vi "Poll Blowers.vi"(8 "error in (no error)":errorcluster, 11 "cRIO-CO2 in":refnum<class "cRIO-CO2.lvclass">) -> (0 "error IO":errorcluster)   [LabVIEW 2015, in "cRIO-Carbondioxide.lvlib" / "cRIO-CO2.lvlib" / "cRIO-CO2.lvclass"]
uses:
  cRIO-CO2.lvclass
  <vilib>/ActorFramework/Actor/Actor.lvclass/Actor.ctl
  <vilib>/ActorFramework/Message Enqueuer/Message Enqueuer.lvclass/Message Enqueuer.ctl
  Blowers Heaters Enumerator.ctl
  cRIO-CO2 Messages/Launch Blower Msg/Launch Blower Msg.lvclass/Launch Blower Msg.ctl
  <vilib>/ActorFramework/Message Enqueuer/Enqueue.vi
  <vilib>/ActorFramework/Message Enqueuer/Init from Existing Queue.vi
  <vilib>/ActorFramework/Message Priority Queue/Priority Enqueue.vi
  cRIO-CO2 Messages/Launch Blower Msg/Launch Blower Msg.lvclass
  <vilib>/ActorFramework/Message Enqueuer/Message Enqueuer.lvclass
  <vilib>/ActorFramework/Actor/Actor.lvclass
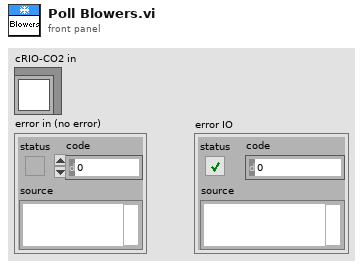
[diagram p1: front panel]
types:
  T1 = typedef "cRIO-Carbondioxide.lvlib/cRIO-CO2.lvlib/cRIO-CO2.lvclass/Blowers Heaters Enumerator.ctl" = enum16{"Tank Blower 1", "Tank Blower 2", "Tank Blower 3", "Tank Blower 4", "Syringe Blower", "Syringe Heater", "Piston Heater", "Undefined"}
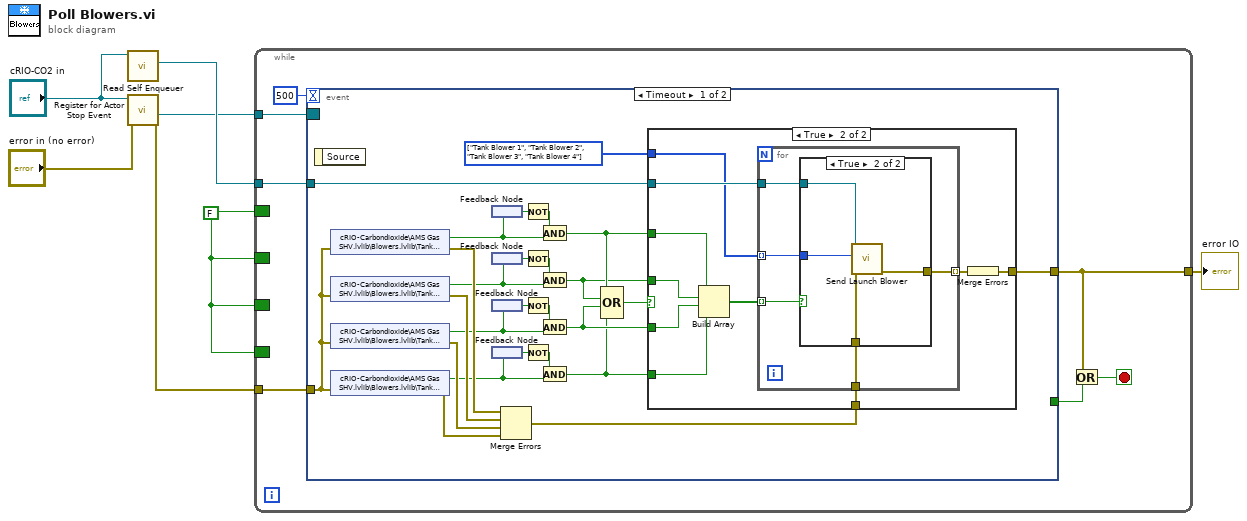
[diagram p0: block diagram]
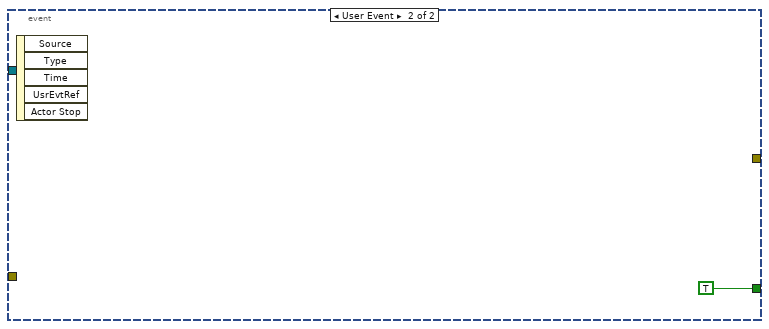
[diagram p4: hidden frame]
diagram:
  w3 = FALSE ("Boolean")
  n1 = call <vilib>:"Read Self Enqueuer.vi"("Actor"="cRIO-CO2 in") -> ("Self Enqueuer"=w5:refnum<class "Message Enqueuer.lvclass">)  [unwired: 10 in]
  n2 = call "Register for Actor Stop Event.vi"("error in (no error)"="error in (no error)", "cRIO-CO2 in"="cRIO-CO2 in") -> ("error out"=w2:errorcluster, "Event Registration Refnum"=w4:refnum<event-registration>)  [unwired: 7 in, 1 out]
  n3 = while {
    tunnel: w5 -> [w14]
    border: w3 -> [_]
    tunnel: w4 -> [w13]
    border: w3 -> [_]
    border: w3 -> [_]
    border: w3 -> [_]
    tunnel: w2 -> [w9]
    tunnel: [w8] -> w1
    stop <- w10 stop-if-true
    n4 = event shown="[0] Timeout" {
      selector: w13 -> [_ _]
      dyn-events: _ -> [_ _]
      timeout: 500 -> [_ _]
      tunnel: w14 -> [w31 _]
      tunnel: [_ TRUE] -> w11
      tunnel: [w24 _] -> w8
      tunnel: w9 -> [w23 _]
      event Timeout {
        w26 = T1[] [enum."Tank Blower 1", enum."Tank Blower 2", enum."Tank Blower 3", enum."Tank Blower 4"] items=["Tank Blower 1", "Tank Blower 2", "Tank Blower 3", "Tank Blower 4", "Syringe Blower", "Syringe Heater", "Piston Heater", "Undefined"]
        n5 = event-data() -> ()  [unwired: 1 in, 1 out]
        n6 = shared-variable "cRIO-Carbondioxide\\AMS Gas SHV.lvlib\\Blowers.lvlib\\Tank Blower 1"(error in=w23) -> (w21:bool, error out=w22:errorcluster)
        n7 = shared-variable "cRIO-Carbondioxide\\AMS Gas SHV.lvlib\\Blowers.lvlib\\Tank Blower 2"(error in=w23) -> (w19:bool, error out=w20:errorcluster)
        n8 = shared-variable "cRIO-Carbondioxide\\AMS Gas SHV.lvlib\\Blowers.lvlib\\Tank Blower 3"(error in=w23) -> (w16:bool, error out=w17:errorcluster)
        n9 = shared-variable "cRIO-Carbondioxide\\AMS Gas SHV.lvlib\\Blowers.lvlib\\Tank Blower 4"(error in=w23) -> (w15:bool, error out=w18:errorcluster)
        n10 = feedback #1() -> (w40:bool)
        n11 = feedback-in #1(w21) -> ()
        n12 = feedback #2() -> (w37:bool)
        n13 = feedback-in #2(w19) -> ()
        n14 = feedback #3() -> (w36:bool)
        n15 = feedback-in #3(w16) -> ()
        n16 = feedback #4() -> (w33:bool)
        n17 = feedback-in #4(w15) -> ()
        n18 = Merge Errors(w22, w20, w17, w18) -> (w25:errorcluster)
        n19 = Not(x=w40) -> (.not. x?=w39:bool)
        n20 = Not(x=w37) -> (.not. x?=w38:bool)
        n21 = Not(x=w36) -> (.not. x?=w35:bool)
        n22 = Not(x=w33) -> (.not. x?=w34:bool)
        n23 = And(x=w39, y=w21) -> (x .and. y?=w30:bool)
        n24 = And(x=w38, y=w19) -> (x .and. y?=w29:bool)
        n25 = And(x=w35, y=w16) -> (x .and. y?=w28:bool)
        n26 = And(x=w34, y=w15) -> (x .and. y?=w27:bool)
        n27 = Compound Arithmetic op=OR(w30, w29, w28, w27) -> (w32:bool)
        n28 = case shown="True" w32 {
          tunnel: w31 -> [_ w46]
          tunnel: w30 -> [_ w51]
          tunnel: w29 -> [_ w50]
          tunnel: w28 -> [_ w49]
          tunnel: w27 -> [_ w48]
          tunnel: w26 -> [_ w45]
          tunnel: w25 -> [w41 w44]
          tunnel: [w41 w42] -> w24
          frame False {
          }
          frame True {
            n29 = Build Array(w51, w50, w49, w48) -> (w47:bool[])
            n30 = for {
              tunnel: w47 -> [w56] mode=indexing
              tunnel: w46 -> [w54]
              tunnel: w45 -> [w55] mode=indexing
              tunnel: w44 -> [w53]
              tunnel: [w52] -> w43 mode=indexing
              n31 = case shown="True" w56 {
                tunnel: w55 -> [_ w60]
                tunnel: w54 -> [_ w61]
                tunnel: w53 -> [w57 w59]
                tunnel: [w57 w58] -> w52
                frame False {
                }
                frame True {
                  n32 = call "Send Launch Blower.vi"("error in (no error)"=w59, "Blower"=w60, "Message Enqueuer"=w61) -> ("error out"=w58:errorcluster)  [unwired: 7 in, 1 out]
                }
              }
            }
            n33 = Merge Errors(w43) -> (w42:errorcluster)
          }
        }
      }
      event User Event {
        n34 = event-data() -> ()  [unwired: 1 in, 5 out]
      }
    }
    n35 = Or(x=w8, y=w11) -> (x .or. y?=w10:bool)
  }
  "error IO" <- w1
